vi "CHD_TRAJECTORY_EXECUTE_ABS.vi"(6 "Pass_Through_Time":dbl=-1.0 format="%33.4f", 8 "Init":bool, 11 "TrajectoryName":string) -> (1 "Complete":bool, 2 "AtReference":bool, 3 "Chassis Velocity Target SI":T1 {"vOmega" format="%10.3f"; "vY" format="%10.3f"; "vX" format="%10.3f"})   [LabVIEW 2019]
uses:
  CHD_TRAJECTORY_GLOBALS.vi
  <vilib>/Rock Robotics/WPI/ThirdParty/JAS_Junk/TrajLib/Trajectory_Library.lvlib
  <vilib>/Rock Robotics/WPI/ThirdParty/ChoreoLib/ChoreoLib.lvlib
  <vilib>/Rock Robotics/WPI/ThirdParty/JAS_Junk/TrajLib/TypeDef/CHASSIS_SPEEDS.ctl
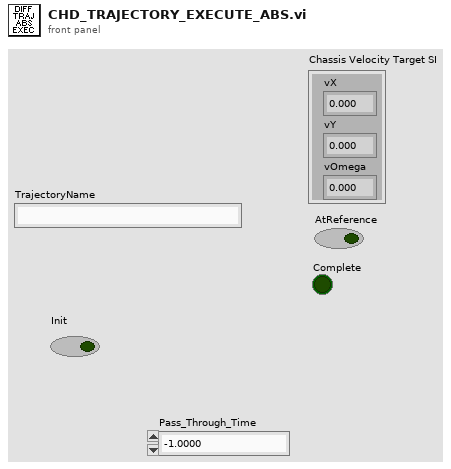
[diagram p1: front panel]
types:
  T1 = typedef "Trajectory_Library.lvlib/CHASSIS_SPEEDS.ctl" = cluster{"vX":dbl, "vY":dbl, "vOmega":dbl}
  T2 = typedef "Trajectory_Library.lvlib/PID_ADV_LIMITS.ctl" = cluster{"MaxInput":dbl, "MinInput":dbl, "Continuous":bool, "MaxOutput":dbl, "MinOutput":dbl}
  T3 = typedef "Trajectory_Library.lvlib/PID_ADV_TUNING.ctl" = cluster{"Kf":dbl, "Kp":dbl, "Ki":dbl, "Kd":dbl, "MaximumIntegral":dbl, "MinimumIntegral":dbl, "Filter Derivative":bool, "IntegralZone":dbl}
  T4 = typedef "Trajectory_Library.lvlib/POSE2D.ctl" = cluster{"TRANSLATION":T5, "ROTATION":T6}
  T5 = typedef "Trajectory_Library.lvlib/TRANSLATION2D.ctl" = cluster{"X":dbl, "Y":dbl}
  T6 = typedef "Trajectory_Library.lvlib/ROTATION2D.ctl" = cluster{"VALUE":dbl, "COS":dbl, "SIN":dbl}
  T7 = typedef "ChoreoLib.lvlib/ChoreoSwerveControlConfig.ctl" = cluster{"X_Adv PID Tuning":T3, "X_Adv PID Limits":T2, "Y_Adv PID Tuning":T3, "Y_Adv PID Limits":T2, "Rot_Adv PID Tuning":T3, "Rot_Adv PID Limits":T2, "X Y Pos Tolerance M":dbl, "Rot Tolerance Deg":dbl, "X Y Vel Tolerance M/S":dbl, "Rot Vel Tolerance Deg/S":dbl}
  T8 = cluster{"X Pos Err M":dbl, "X Vel Err M/S":dbl, "Y Pos Err M":dbl, "Y Vel Err M/S":dbl, "Rot Pos Err Deg":dbl, "Rot Vel Err Deg/Sec":dbl}
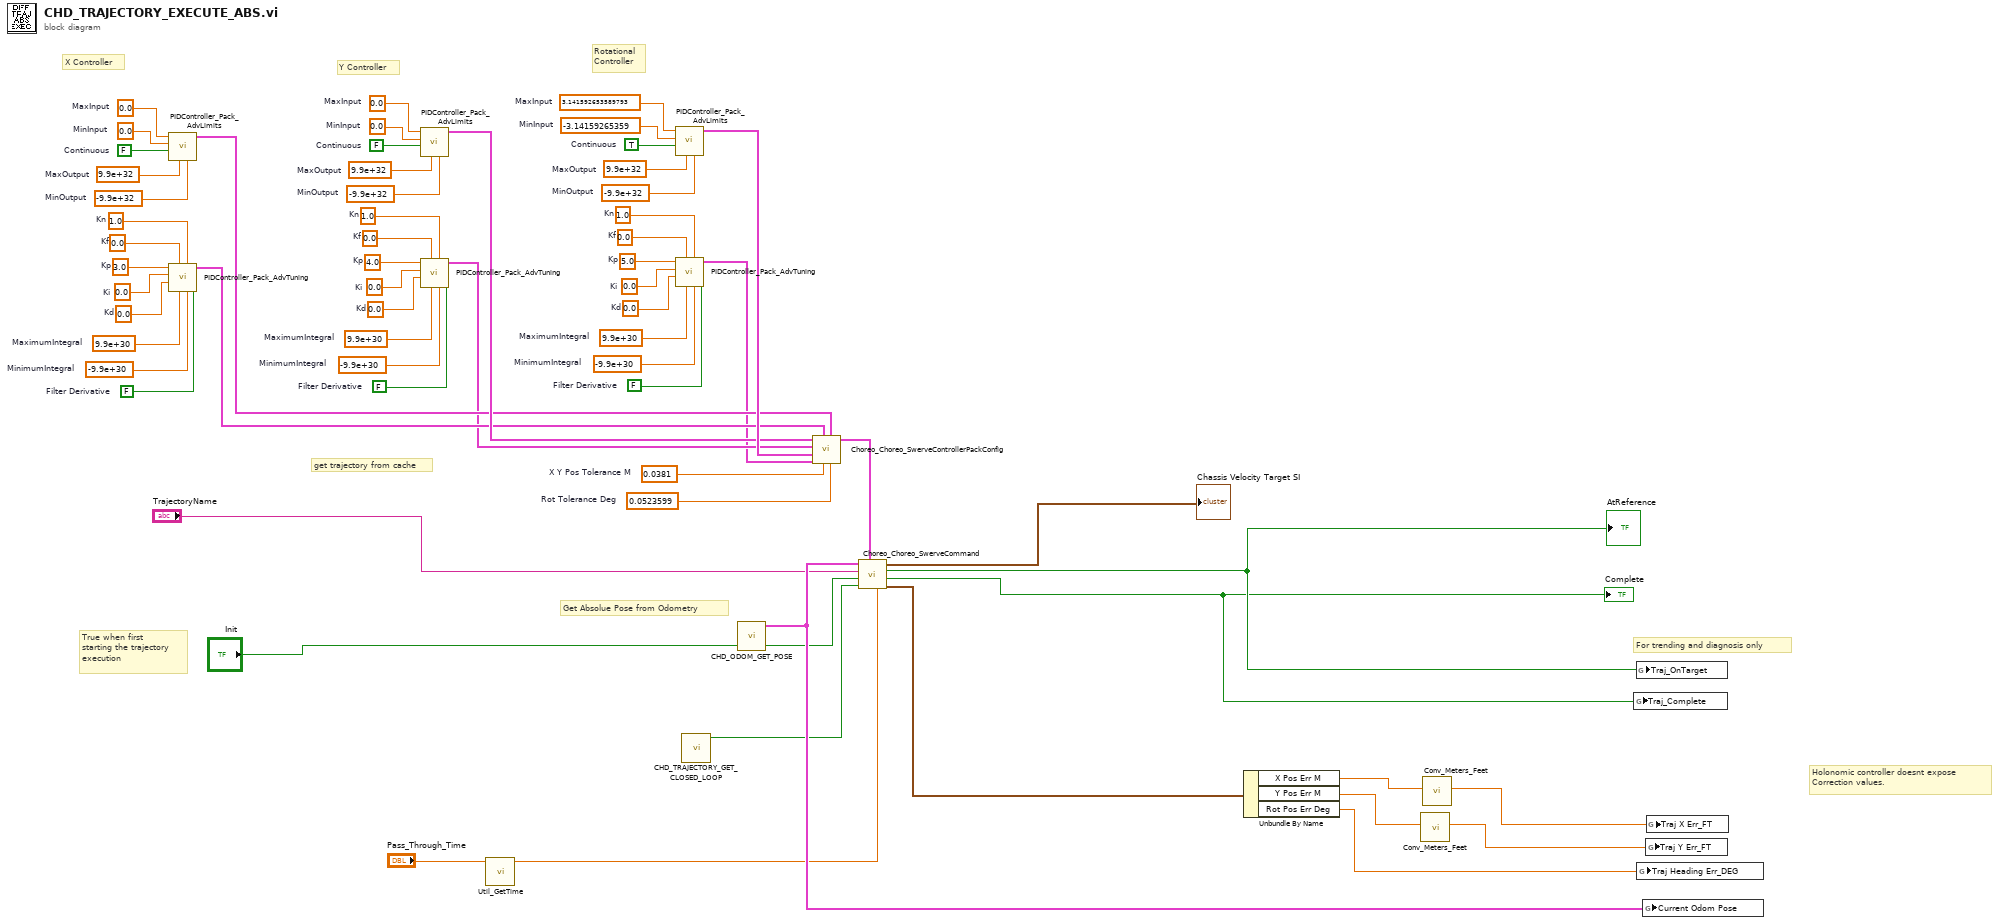
[diagram p0: block diagram]
diagram:
  w63 = 0.0523599  # Rot Tolerance Deg
  w62 = 0.0381  # X Y Pos Tolerance M
  w43 = 1.0  # Kn
  w44 = 5.0  # Kp
  w45 = 0.0  # Ki
  w46 = 0.0  # Kd
  w47 = 0.0  # Kf
  w48 = 9.9e+30  # MaximumIntegral
  w49 = -9.9e+30  # MinimumIntegral
  w50 = FALSE  # Filter Derivative
  w52 = -3.14159265359  # MinInput
  w53 = TRUE  # Continuous
  w54 = 9.9e+32  # MaxOutput
  w51 = -9.9e+32  # MinOutput
  w55 = 3.141592653589793  # MaxInput
  w30 = 1.0  # Kn
  w31 = 4.0  # Kp
  w32 = 0.0  # Ki
  w33 = 0.0  # Kd
  w34 = 0.0  # Kf
  w35 = 9.9e+30  # MaximumIntegral
  w36 = -9.9e+30  # MinimumIntegral
  w37 = FALSE  # Filter Derivative
  w39 = 0.0  # MinInput
  w40 = FALSE  # Continuous
  w41 = 9.9e+32  # MaxOutput
  w38 = -9.9e+32  # MinOutput
  w42 = 0.0  # MaxInput
  w17 = 1.0  # Kn
  w18 = 3.0  # Kp
  w19 = 0.0  # Ki
  w20 = 0.0  # Kd
  w21 = 0.0  # Kf
  w22 = 9.9e+30  # MaximumIntegral
  w23 = -9.9e+30  # MinimumIntegral
  w24 = FALSE  # Filter Derivative
  w26 = 0.0  # MinInput
  w27 = FALSE  # Continuous
  w28 = 9.9e+32  # MaxOutput
  w25 = -9.9e+32  # MinOutput
  w29 = 0.0  # MaxInput
  # "get trajectory from cache"
  # "Rotational\nController"
  # "Y Controller"
  # "X Controller"
  # "True when first\nstarting the trajectory\nexecution"
  # "Holonomic controller doesnt expose\nCorrection values."
  # "For trending and diagnosis only"
  # "Get Absolue Pose from Odometry"
  n1 = call <vilib>:"PIDController_Pack_AdvLimits.vi"("MinOutput"=w25, "MaxOutput"=w28, "Continuous"=w27, "MinInput"=w26, "MaxInput"=w29) -> ("Adv PID Limits"=w59:T2)  [unwired: 6 in]
  n2 = call <vilib>:"PIDController_Pack_AdvTuning.vi"("Filter Derivative"=w24, "MinimumIntegral"=w23, "Kn"=w17, "MaximumIntegral"=w22, "Kf"=w21, "Kd"=w20, "Ki"=w19, "Kp"=w18) -> ("Adv PID Tuning"=w58:T3)  [unwired: 3 in]
  n3 = call <vilib>:"PIDController_Pack_AdvLimits.vi"("MinOutput"=w38, "MaxOutput"=w41, "Continuous"=w40, "MinInput"=w39, "MaxInput"=w42) -> ("Adv PID Limits"=w60:T2)  [unwired: 6 in]
  n4 = call <vilib>:"PIDController_Pack_AdvTuning.vi"("Filter Derivative"=w37, "MinimumIntegral"=w36, "Kn"=w30, "MaximumIntegral"=w35, "Kf"=w34, "Kd"=w33, "Ki"=w32, "Kp"=w31) -> ("Adv PID Tuning"=w57:T3)  [unwired: 3 in]
  n5 = call <vilib>:"Util_GetTime.vi"("Pass_Through_Time"="Pass_Through_Time") -> ("FPGA_Time_Seconds"=w9:dbl)  [unwired: 8 in, 2 out]
  n6 = call <vilib>:"PIDController_Pack_AdvLimits.vi"("MinOutput"=w51, "MaxOutput"=w54, "Continuous"=w53, "MinInput"=w52, "MaxInput"=w55) -> ("Adv PID Limits"=w61:T2)  [unwired: 6 in]
  n7 = call <vilib>:"PIDController_Pack_AdvTuning.vi"("Filter Derivative"=w50, "MinimumIntegral"=w49, "Kn"=w43, "MaximumIntegral"=w48, "Kf"=w47, "Kd"=w46, "Ki"=w45, "Kp"=w44) -> ("Adv PID Tuning"=w56:T3)  [unwired: 3 in]
  n8 = call "CHD_TRAJECTORY_GET_CLOSED_LOOP.vi"() -> ("AUTO_CLOSED_LOOP"=w14:bool)  [unwired: 11 in]
  n9 = call "CHD_ODOM_GET_POSE.vi"() -> ("Absolute Odometry Pose"=w15:T4)  [unwired: 11 in]
  n10 = call <vilib>:"Choreo_Choreo_SwerveControllerPackConfig.vi"("Rot Tolerance Deg"=w63, "X_Adv PID Limits"=w59, "X Y Pos Tolerance M"=w62, "X_Adv PID Tuning"=w58, "Rot_Adv PID Tuning"=w56, "Rot_Adv PID Limits"=w61, "Y_Adv PID Tuning"=w57, "Y_Adv PID Limits"=w60) -> ("ChoreoSwerveControlConfig"=w16:T7)  [unwired: 3 in]
  n11 = call <vilib>:"Choreo_Choreo_SwerveCommand.vi"("Pass_Through_Time"=w9, "ChoreoSwerveControlConfig"=w16, "Auto"=w14, "Initialize"="Init", "TrajectoryName"="TrajectoryName", "Current Position"=w15) -> ("Ctrl Info"=w6:T8, "Complete"=w11:bool, "On Target"=w12:bool, "Chassis Speed Dmd"=→"Chassis Velocity Target SI":T1)  [unwired: 2 in]
  "AtReference" <- w12
  "Complete" <- w11
  n12 = Unbundle By Name(w6) -> ("X Pos Err M"=w5:dbl, "Y Pos Err M"=w4:dbl, "Rot Pos Err Deg"=w3:dbl)
  n13 = call <vilib>:"Conv_Meters_Feet.vi"("Meters"=w4) -> ("Feet"=w8:dbl)  [unwired: 10 in]
  n14 = call <vilib>:"Conv_Meters_Feet.vi"("Meters"=w5) -> ("Feet"=w7:dbl)  [unwired: 10 in]
  n15 = global write "CHD_TRAJECTORY_GLOBALS.vi" "Traj_Complete"(w11) -> ()
  n16 = global write "CHD_TRAJECTORY_GLOBALS.vi" "Traj_OnTarget"(w12) -> ()
  n17 = global write "CHD_TRAJECTORY_GLOBALS.vi" "Traj Heading Err_DEG"(w3) -> ()
  n18 = global write "CHD_TRAJECTORY_GLOBALS.vi" "Current Odom Pose"(w15) -> ()
  n19 = global write "CHD_TRAJECTORY_GLOBALS.vi" "Traj Y Err_FT"(w8) -> ()
  n20 = global write "CHD_TRAJECTORY_GLOBALS.vi" "Traj X Err_FT"(w7) -> ()
